vi "Create diagram name.vi"(11 "Working Path":path) -> (3 "appended path":path)   [LabVIEW 2020, in "SimpleDependencyInspector.lvlib"]
uses:
  SimpleDependencyInspector.lvlib
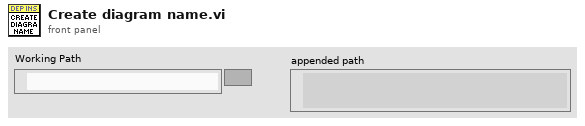
[diagram p1: front panel]
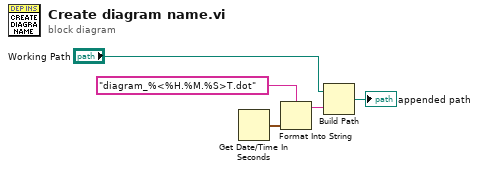
[diagram p0: block diagram]
diagram:
  n1 = Get Date/Time In Seconds() -> (seconds since 1Jan1904=w5:timestamp)
  n2 = Format Into String(format string="diagram_%<%H.%M.%S>T.dot", w5) -> (resulting string=w2:string)  [unwired: 2 in, 1 out]
  n3 = Build Path(base path="Working Path", name or relative path=w2) -> (appended path=→"appended path":path)
